vi "PythonIDE.vi"(7 "Python version":string="3.9", 9 "Processor":u16(ring) items=["SPIKE", "Pi", "Pi_ssh"], 11 "Port":string) -> ()   [LabVIEW 2020]
uses:
  <vilib>/event_ctls.llb/eventvkey.ctl
  <vilib>/Utility/miscctls.llb/LVSelectionTypeDef.ctl
  Comm_Global.vi
  <vilib>/Platform/browser.llb/Open URL in Default Browser (string).vi
panel:
  out "Text.Scroll Position":u32
  in  "Format":T1(ring)
  in  "Name":string="main.py"
  in  "Spaces":bool
  out "Shift":bool
  in  "Explorer":u16(ring) items=["Explore...", "Arm", "Backpack", "Image", "Motors", "Pinouts", "Scope", "Spatial Toolbox", "Twin"]
  in  "reconnect":bool
  out "VKey":T2
  in  "Browser":bool
  out "error IO":errorcluster
  in  "Tree":string(tree)
  in  "CtrlE":bool
  in  "Font Size":u32=12
  in  "run":bool
  in  "Save SPIKE":bool
  out "Script":string
  in  "Python Code":string
  out "Line #":string
  out "Buffer":i32(slide) scale=0.0..100000.0
  out "Graph":dbl[](graph)
  out "JPG":picture
  out "Chart":dbl[](graph)
  out "Console":string
  out "Path":path
  in  "Clear":bool
  in  "Ctrl C":bool
  in  "Save Log":bool
  in  "stop":bool
  # "PyVIEW IDE\nversion 0.1b21"
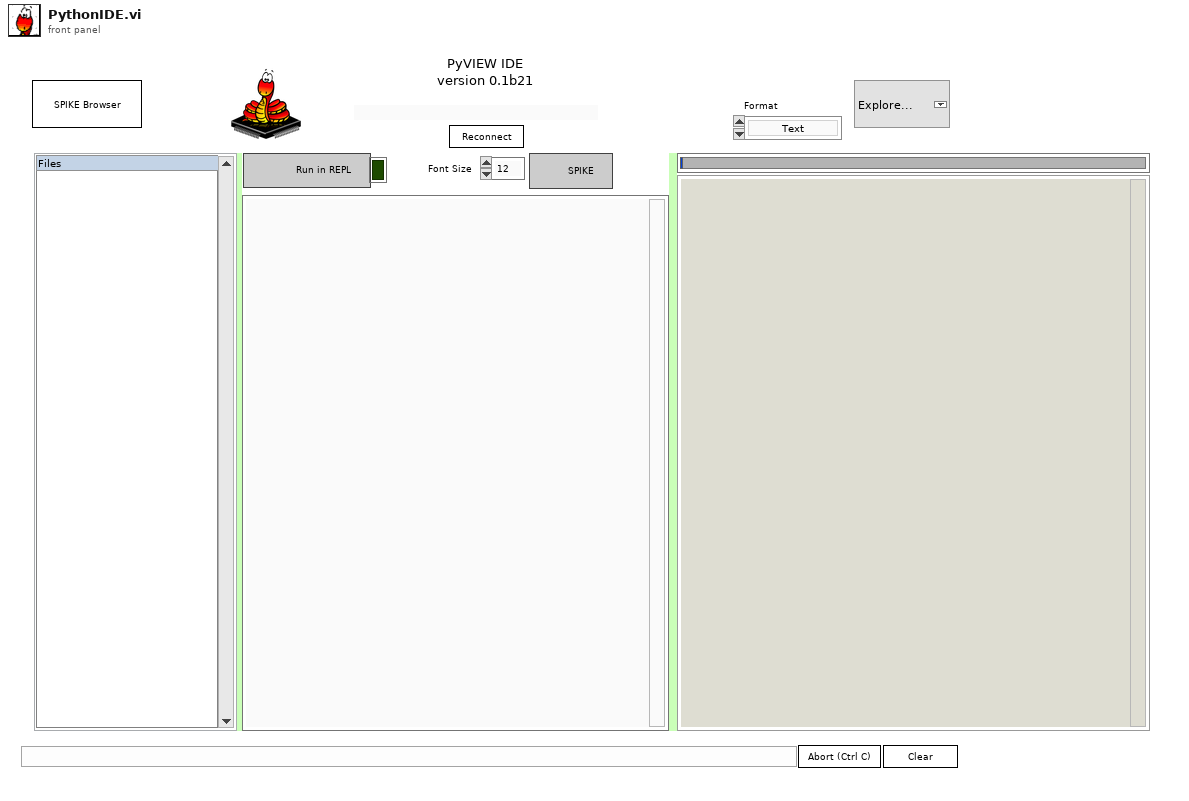
[diagram p1: front panel]
types:
  T1 = enum16{"Text", "Chart", "Waveforms", "JPEG", "Split View"}
  T2 = typedef "eventvkey.ctl" = enum16{"ASCII", "Enter", "Return", "Shift", "Ctrl", "Alt", "Cmd", "Opt", "Caps", "NumLock", "Clear", "Break", "Up", "Down", "Left", "Right", "Insert", "Delete", "Home", "End", "PageUp", "PageDown", "Escape", "Help", "Pause", "ScrollLock", "F1", "F2", "F3", "F4", "F5", "F6", "F7", "F8", "F9", "F10", "F11", "F12", "F13", "F14", "F15", "F16", "F17", "F18", "F19", "F20", "F21", "F22", "F23", "F24", "Play", "VolumeUp", "VolumeDown", "Mute", "Two Byte Char"}
  T3 = typedef "PythonCtrl.ctl" = cluster{"session":refnum<k35>, "PyPath":path, "Processor":T4}
  T4 = typedef "Processors.ctl" = enum16{"SPIKE", "Pi", "Pi_ssh", "OpenMV"}
  T5 = enum8{"Enabled", "Disabled", "Disabled and Grayed Out"}
  T6 = typedef "LVSelectionTypeDef.ctl" = cluster{"Selection Start":u32, "Selection End":u32}
  T7 = enum16{"Not data", "single values", "XY pairs", "Arrays"}
  T8 = typedef "LVPoint32TypeDef.ctl" = cluster{"Horizontal":i32, "Vertical":i32}
  T9 = typedef "Preferences.ctl" = cluster{"python":string, "arduino15":path, "arduino Lib":path, "pythonCodes":cluster{"pythonCode":path, "Color":u32}[], "FontSize":u8, "Text Colors":cluster{"Quote":u32, "function":u32, "Python":u32, "Comment":u32, "Triple Quote":u32, "Text":u32}, "Raspberry Pi":cluster{"Username":string, "password":string}}
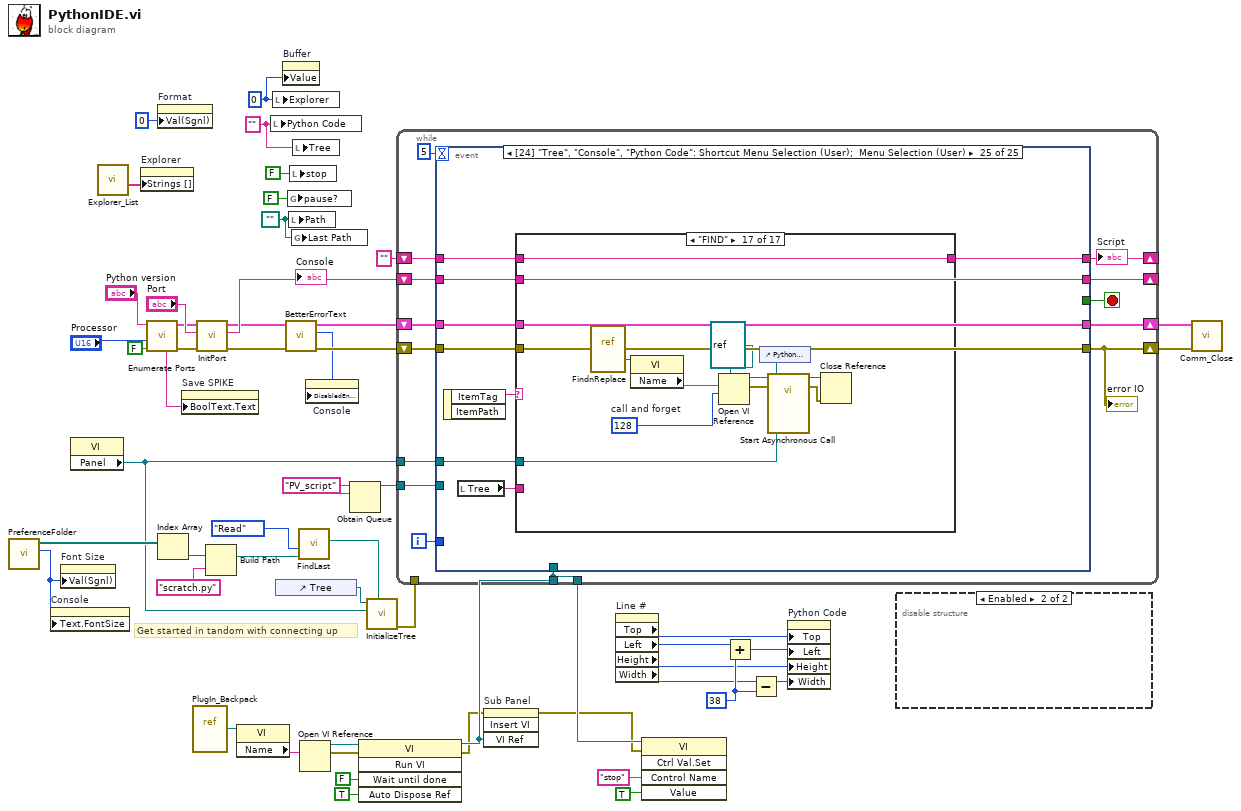
[diagram p0: block diagram]
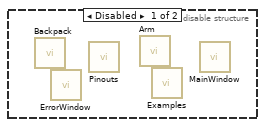
[diagram p2: hidden frame]
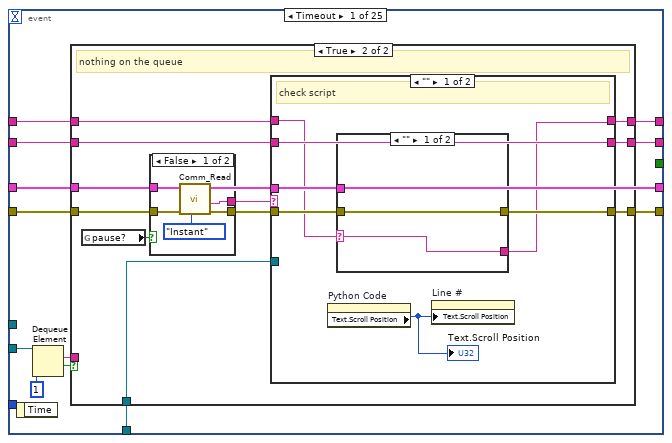
[diagram p3: hidden frame]
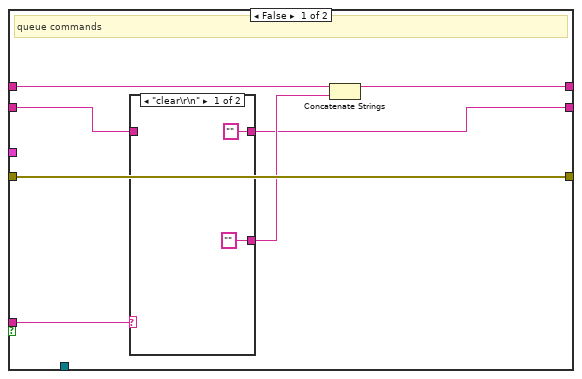
[diagram p4: hidden frame]
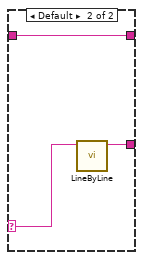
[diagram p5: hidden frame]
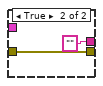
[diagram p6: hidden frame]
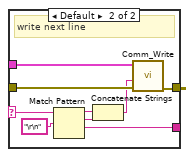
[diagram p7: hidden frame]
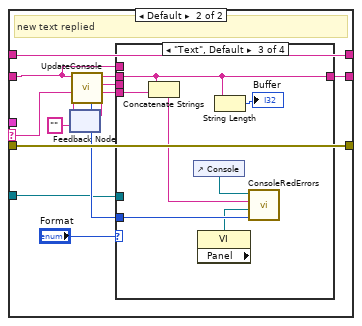
[diagram p8: hidden frame]
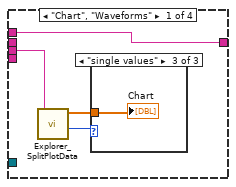
[diagram p9: hidden frame]
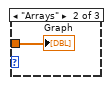
[diagram p11: hidden frame]
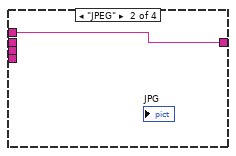
[diagram p12: hidden frame]
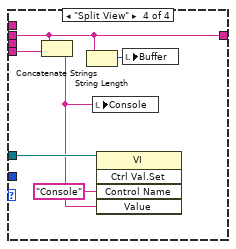
[diagram p13: hidden frame]
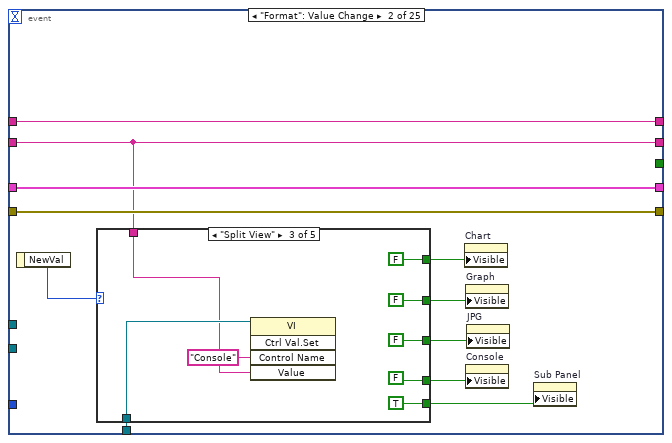
[diagram p14: hidden frame]
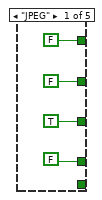
[diagram p15: hidden frame]
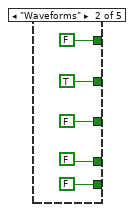
[diagram p16: hidden frame]
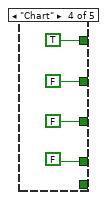
[diagram p17: hidden frame]
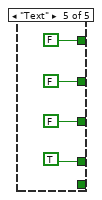
[diagram p18: hidden frame]
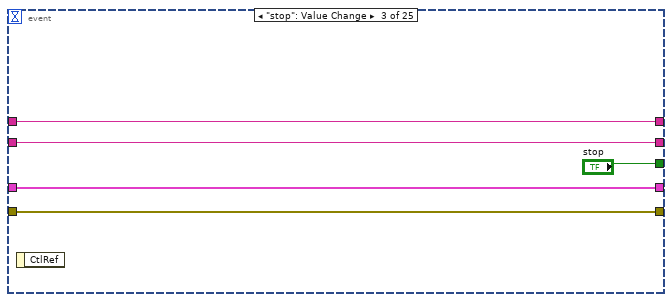
[diagram p19: hidden frame]
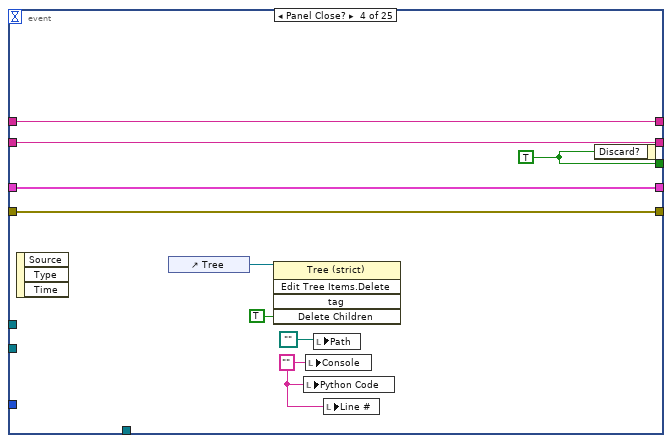
[diagram p20: hidden frame]
diagram:
  w26 = 38 ("y")
  w18 = path "" ("Path")
  w29 = 0
  w43 = "PV_script" ("name (unnamed)")
  w46 = "" ("Python Code")
  # "Get started in tandom with connecting up"
  n1 = call "PreferenceFolder.vi"() -> ("FontSize"=w16:u8, "pythonCodes"=w34:path[])  [unwired: 6 in, 4 out]
  n2 = property on="Console" class="Str"("Text.FontSize"=w16) -> ()  [unwired: 2 in, 2 out]
  n3 = property on="Font Size" class="DigNum (strict)"("Val(Sgnl)"=w16) -> ()  [unwired: 2 in, 2 out]
  n4 = property class="VI"() -> ("Panel"=w1:refnum<vi>)  [unwired: 2 in, 2 out]
  n5 = call "Explorer_List.vi"() -> ("Options"=w41:string[])  [unwired: 9 in, 2 out]
  n6 = property on="Explorer" class="Ring (strict)"("Strings []"=w41) -> ()  [unwired: 2 in, 2 out]
  n7 = call "Enumerate Ports.vi"("list?"=FALSE, "Processor"="Processor", "Python version"="Python version") -> ("error out"=w48:errorcluster, "Python"=w49:T3, "name"=w40:string)  [unwired: 4 in, 2 out]
  n8 = property on="Format" class="Enum (strict)"("Val(Sgnl)"=0) -> ()  [unwired: 2 in, 2 out]
  n9 = Index Array(array=w34) -> (element=w33:path)  [unwired: 1 in]
  n10 = property on="Save SPIKE" class="Bool"("BoolText.Text"=w40) -> ()  [unwired: 2 in, 2 out]
  n11 = vi-ref "PlugIn_Backpack.vi"() -> (w9:refnum<vi>)
  n12 = call "InitPort.vi"("error in (no error)"=w48, "Port"="Port", "Python"=w49) -> ("error out"=w15:errorcluster, "Console"=w36:string, "Python out"=w28:T3)  [unwired: 6 in]
  "Console" <- w36
  n13 = Build Path(base path=w33, name or relative path="scratch.py" ("Python Code")) -> (appended path=w32:path)
  n14 = property class="VI"(reference=w9) -> ("Name"=w7:string)  [unwired: 1 in, 2 out]
  n15 = local write "Python Code"(w46) -> ()
  n16 = local write "Explorer"(w29) -> ()
  n17 = control-ref of="Tree"() -> (w38:refnum<vi>)
  n18 = property on="Buffer" class="Slide (strict)"("Value"=w29) -> ()  [unwired: 2 in, 2 out]
  n19 = call "BetterErrorText.vi"("error in (no error)"=w15, "Python"=w28) -> ("Disabled"=w14:T5, "Python out"=w19:T3)  [unwired: 8 in]
  n20 = global write "Comm_Global.vi" "pause?"(FALSE ("pause?")) -> ()
  n21 = local write "Path"(w18) -> ()
  n22 = local write "stop"(FALSE ("stop")) -> ()
  n23 = global write "Comm_Global.vi" "Last Path"(w18) -> ()
  n24 = local write "Tree"(w46) -> ()
  n25 = call "FindLast.vi"("default"=w32, "Task"=enum16{"Save", "Read"}."Read") -> ("path"=w31:path)  [unwired: 9 in]
  n26 = Open VI Reference(vi path=w7) -> (vi reference=w11:refnum<vi>, error out=w10:errorcluster)  [unwired: 5 in]
  n27 = property on="Console" class="Str"("DisabledEnum"=w14) -> ()  [unwired: 2 in, 2 out]
  n28 = Obtain Queue(name (unnamed)=w43, element data type=w43) -> (queue out=w42:refnum<queue>)  [unwired: 3 in, 2 out]
  n29 = invoke class="VI" method="Run VI"(reference=w11, error in=w10, "Wait until done"=FALSE ("Wait Until Done"), "Auto Dispose Ref"=TRUE ("Auto Dispose Reference")) -> (reference out=w8:refnum<vi>, error out=w3:errorcluster)  [unwired: 1 in, 3 out]
  n30 = call "InitializeTree.vi"("Selected File"=w31, "Panel"=w1, "TreeControl in"=w38) -> ("error out"=w20:errorcluster)  [unwired: 8 in]
  n31 = while {
    shift-right: [w65] -> _
    shift-left: w36 -> [w66]
    shift-right: [w54] -> w44
    shift-left: w15 -> [w62]
    tunnel: w1 -> [w61]
    shift-right: [w59] -> _
    shift-left: "" -> [w60]
    tunnel: w42 -> [w57]
    shift-right: [w56] -> _
    shift-left: w19 -> [w58]
    tunnel: w20 -> [_]
    tunnel: w8 -> [w53]
    tunnel: [w53] -> w5
    i -> [w55]
    stop <- w64 stop-if-true
    n32 = event shown="[24] \"Tree\", \"Console\", \"Python Code\": Shortcut Menu Selection (User);  Menu Selection (User)" {
      selector: _ -> [_ _ _ _ _ _ _ _ _ _ _ _ _ _ _ _ _ _ _ _ _ _ _ _ _]
      dyn-events: _ -> [_ _ _ _ _ _ _ _ _ _ _ _ _ _ _ _ _ _ _ _ _ _ _ _ _]
      timeout: 5 -> [_ _ _ _ _ _ _ _ _ _ _ _ _ _ _ _ _ _ _ _ _ _ _ _ _]
      tunnel: w58 -> [w68 w171 w197 w203 w219 w224 w240 w324 w329 w338 w359 w379 w394 w407 w419 w437 w461 w472 w480 w487 w497 w503 w517 w526 w537]
      tunnel: w66 -> [w78 w161 w200 w210 w222 w231 w255 w327 w334 w347 w360 w385 w405 w411 w420 w442 w464 w475 _ w489 w500 w512 w523 w532 w536]
      tunnel: [w77 w161 w200 w210 w222 w231 w255 w327 w334 w347 w360 w385 w405 w411 w420 w442 w464 w475 w485 w489 w500 w512 w523 w532 w536] -> w65
      tunnel: [_ _ "stop" w207 _ _ _ _ _ _ _ _ _ _ _ _ _ _ _ _ _ _ _ _ _] -> w64
      tunnel: w62 -> [w73 w170 w199 w209 w221 w230 w249 w326 w333 w346 w355 w384 w406 w412 w418 w440 w462 w473 w486 w493 w502 w514 w525 w534 w539]
      tunnel: [w76 w170 w199 w209 w221 w230 w250 w326 w331 w346 w361 w384 w406 w412 w417 w440 w462 w473 w486 w493 w502 w514 w525 w534 w539] -> w54
      tunnel: w61 -> [_ _ _ _ _ _ _ _ _ w345 _ _ _ _ _ _ w460 _ _ _ _ _ _ _ w542]
      tunnel: [w75 w169 w198 w208 w220 w228 w246 w328 "" w344 w362 w386 w404 w410 w413 w441 w463 w474 w482 w492 w501 w513 w524 w533 w535] -> w59
      tunnel: w60 -> [w74 w169 w198 w208 w220 w229 w247 w328 _ w344 w362 w386 w404 w410 w414 w441 w463 w474 w484 w492 w501 w513 w524 w533 w538]
      tunnel: w57 -> [w72 _ _ _ _ _ _ _ _ _ _ _ _ _ _ _ _ _ _ _ _ _ _ _ _]
      tunnel: [w68 w171 w197 w203 w219 w224 w240 w324 w329 w338 w359 w379 w394 w407 w416 w437 w461 w472 w480 w487 w497 w503 w517 w526 w537] -> w56
      tunnel: w55 -> [_ _ _ _ _ _ _ _ _ w335 _ _ _ _ _ _ _ _ _ _ _ _ _ _ _]
      tunnel: w53 -> [w67 w162 _ _ _ _ _ _ _ _ _ _ _ _ _ _ _ _ _ _ _ _ _ _ _]
      event Timeout {
        n33 = event-data() -> ()  [unwired: 1 in, 1 out]
        n34 = Dequeue Element(queue=w72, timeout in ms (-1)=1) -> (element=w69:string, timed out?=w70:bool)  [unwired: 1 in, 2 out]
        n35 = case shown="True" w70 {
          tunnel: w78 -> [w79 w92]
          tunnel: [w80 w94] -> w77
          tunnel: [w85 w101] -> w76
          tunnel: [w83 w100] -> w75
          tunnel: w74 -> [w84 w99]
          tunnel: w73 -> [w85 w98]
          tunnel: w68 -> [_ w96]
          tunnel: w69 -> [w81 _]
          tunnel: w67 -> [_ w91]
          frame False {
            # "queue commands"
            n36 = case shown="\"clear\\r\\n\"" w81 {
              selector: w81 -> [_ w88]
              tunnel: ["" ("result string") w90] -> w82
              tunnel: ["" ("Console") w89] -> w80
              tunnel: w79 -> [_ w89]
              frame "clear\r\n" {
              }
              frame Default {
                n37 = call "LineByLine.vi"("Python Code"=w88) -> ("result string"=w90:string)  [unwired: 10 in]
              }
            }
            n38 = Concatenate Strings(w84, w82) -> (w83:string)
          }
          frame True {
            # "nothing on the queue"
            n39 = global read "Comm_Global.vi" "pause?"() -> (w95:bool)
            n40 = case shown="False" w95 {
              tunnel: w98 -> [w106 w108]
              tunnel: [w105 "" ("Text read")] -> w93
              tunnel: [w104 w108] -> w97
              tunnel: w96 -> [w103 _]
              frame False {
                n41 = call "Comm_Read.vi"("Task"=enum16{"Instant", "All"}."Instant", "error in (no error)"=w106, "Python"=w103) -> ("error out"=w104:errorcluster, "Text read"=w105:string)  [unwired: 7 in]
              }
              frame True {
              }
            }
            n42 = case shown="\"\"" w93 {
              selector: w93 -> [_ w133]
              tunnel: w92 -> [w112 w128]
              tunnel: w97 -> [w115 w140]
              tunnel: [w114 w140] -> w101
              tunnel: w99 -> [w111 w139]
              tunnel: [w110 w139] -> w100
              tunnel: w96 -> [w113 _]
              tunnel: [w112 w129] -> w94
              tunnel: w91 -> [_ w127]
              frame "" {
                # "check script"
                n43 = property on="Python Code" class="Str"() -> ("Text.Scroll Position"=w109:u32)  [unwired: 2 in, 2 out]
                "Text.Scroll Position" <- w109
                n44 = case shown="\"\"" w111 {
                  selector: w111 -> [w116 w118]
                  tunnel: [w116 w126] -> w110
                  tunnel: w115 -> [w117 w122]
                  tunnel: [w117 w121] -> w114
                  tunnel: w113 -> [_ w119]
                  frame "" {
                  }
                  frame Default {
                    # "write next line"
                    n45 = Match Pattern(string=w118, regular expression="\r\n") -> (before substring=w124:string, match substring=w123:string, after substring=w126:string)  [unwired: 1 in, 1 out]
                    n46 = Concatenate Strings(w124, w123) -> (w120:string)
                    n47 = call "Comm_Write.vi"("error in (no error)"=w122, "Text to write"=w120, "Python"=w119) -> ("error out"=w121:errorcluster)  [unwired: 8 in]
                  }
                }
                n48 = property on="Line #" class="Str"("Text.Scroll Position"=w109) -> ()  [unwired: 2 in, 2 out]
              }
              frame Default {
                # "new text replied"
                n49 = feedback #1("" ("Left over raw")) -> (w137:string)
                n50 = call "UpdateConsole.vi"("from last time raw"=w137, "New Text"=w133, "Console"=w128) -> ("Left over raw"=w138:string, "left over fixed"=w131:string, "LastFullLine"=w132:string, "Console Out"=w130:string, "cursor out"=w135:i32)  [unwired: 4 in]
                n51 = feedback-in #1(w138) -> ()
                n52 = case shown="\"Text\", Default" "Format" {
                  tunnel: w135 -> [_ _ w154 _]
                  tunnel: w132 -> [w144 _ _ _]
                  tunnel: w130 -> [_ _ w150 w159]
                  tunnel: w131 -> [_ _ w152 w160]
                  tunnel: [w141 w147 w150 w159] -> w129
                  tunnel: w128 -> [w141 w147 _ _]
                  tunnel: w127 -> [_ _ _ w156]
                  frame "Chart", "Waveforms" {
                    n53 = call "Explorer_SplitPlotData.vi"("Value"=w144) -> ("Data type"=w142:T7, "Array"=w143:dbl[])  [unwired: 9 in]
                    n54 = case shown="\"single values\"" w142 {
                      tunnel: w143 -> [_ w145 w146]
                      frame Default {
                      }
                      frame "Arrays" {
                        "Graph" <- w145
                      }
                      frame "single values" {
                        "Chart" <- w146
                      }
                    }
                  }
                  frame "JPEG" {
                  }
                  frame "Text", Default {
                    n55 = Concatenate Strings(w150, w152) -> (w151:string)
                    n56 = control-ref of="Console"() -> (w149:refnum<vi>)
                    n57 = property class="VI"() -> ("Panel"=w148:refnum<vi>)  [unwired: 2 in, 2 out]
                    n58 = String Length(string=w150) -> (length=→"Buffer":i32)
                    n59 = call "ConsoleRedErrors.vi"("Text.Selection:End"=w154, "Front Panel"=w148, "Console in"=w151, "String in"=w149) -> ()  [unwired: 6 in, 2 out]
                  }
                  frame "Split View" {
                    n60 = Concatenate Strings(w159, w160) -> (w155:string)
                    n61 = String Length(string=w159) -> (length=w158:i32)
                    n62 = local write "Console"(w155) -> ()
                    n63 = invoke class="VI" method="Ctrl Val.Set"(reference=w156, "Control Name"="Console", "Value"=w155) -> ()  [unwired: 2 in, 5 out]
                    n64 = local write "Buffer"(w158) -> ()
                  }
                }
              }
            }
          }
        }
      }
      event "Format": Value Change {
        n65 = event-data() -> ("NewVal"=w168:T1)  [unwired: 1 in]
        n66 = case shown="\"Split View\"" w168 {
          tunnel: [TRUE ("Visible") FALSE ("Visible") FALSE ("Visible") FALSE ("Visible") FALSE ("Visible")] -> w167
          tunnel: [FALSE ("Visible") TRUE ("Visible") FALSE ("Visible") FALSE ("Visible") FALSE ("Visible")] -> w166
          tunnel: [FALSE ("Visible") FALSE ("Visible") FALSE ("Visible") TRUE ("Visible") FALSE ("Visible")] -> w165
          tunnel: [FALSE ("Visible") FALSE ("Visible") FALSE ("Visible") FALSE ("Visible") TRUE ("Visible")] -> w164
          tunnel: [_ FALSE ("Visible") TRUE ("Visible") _ _] -> w163
          tunnel: w162 -> [_ _ w182 _ _]
          tunnel: w161 -> [_ _ w181 _ _]
          frame "JPEG" {
          }
          frame "Waveforms" {
          }
          frame "Split View" {
            n67 = invoke class="VI" method="Ctrl Val.Set"(reference=w182, "Control Name"="Console", "Value"=w181) -> ()  [unwired: 2 in, 5 out]
          }
          frame "Chart" {
          }
          frame "Text" {
          }
        }
        n68 = property on="Chart" class="WFChart (strict)"("Visible"=w165) -> ()  [unwired: 2 in, 2 out]
        n69 = property on="Graph" class="WFGraph (strict)"("Visible"=w166) -> ()  [unwired: 2 in, 2 out]
        n70 = property on="Console" class="Str"("Visible"=w164) -> ()  [unwired: 2 in, 2 out]
        n71 = property on="JPG" class="Pict"("Visible"=w167) -> ()  [unwired: 2 in, 2 out]
        n72 = property on="Sub Panel" class="SubPnl"("Visible"=w163) -> ()  [unwired: 2 in, 2 out]
      }
      event "stop": Value Change {
        n73 = event-data() -> ()  [unwired: 1 in, 1 out]
      }
      event Panel Close? {
        w202 = "" ("source")
        w207 = TRUE ("stop")
        n74 = event-data() -> ()  [unwired: 1 in, 3 out]
        n75 = control-ref of="Tree"() -> (w206:refnum<vi>)
        n76 = invoke on="Invoke Node" class="Tree (strict)" method="Edit Tree Items.Delete"(reference=w206, "Delete Children"=TRUE ("Delete Children?")) -> ()  [unwired: 3 in, 5 out]
        n77 = local write "Python Code"(w202) -> ()
        n78 = local write "Console"(w202) -> ()
        n79 = local write "Path"(path "") -> ()
        n80 = local write "Line #"(w202) -> ()
        n81 = event-data("Discard?"=w207) -> ()  [unwired: 1 in, 1 out]
      }
      event Pane Size; Panel Resize {
        w213 = 38 ("y")
        n82 = event-data() -> ()  [unwired: 1 in, 5 out]
        n83 = property on="Line #" class="Str"() -> ("Top"=w216:i32, "Left"=w218:i32, "Height"=w215:u32, "Width"=w214:u32)  [unwired: 2 in, 2 out]
        n84 = local read "Text.Scroll Position"() -> (w211:u32)
        n85 = Add(x=w218, y=w213) -> (x+y=w217:i32)
        n86 = Subtract(x=w214, y=w213) -> (x-y=w212:u32)
        n87 = property on="Python Code" class="Str"("Text.Scroll Position"=w211, "Top"=w216, "Left"=w217, "Height"=w215, "Width"=w212) -> ()  [unwired: 2 in, 2 out]
      }
      event "run": Value Change {
        n88 = event-data() -> ()  [unwired: 1 in, 1 out]
        n89 = local read "Processor"() -> (w225:u16)
        n90 = case shown="False" "CtrlE" {
          tunnel: [w234 w237] -> w227
          tunnel: "Python Code" -> [w233 w238]
          tunnel: w225 -> [w232 _]
          frame False {
            n91 = call "LineByLine.vi"("Processor"=w232, "Python Code"=w233) -> ("result string"=w234:string)  [unwired: 9 in]
          }
          frame True {
            n92 = Concatenate Strings("\u0005" ("string"), w238, "\u0004" ("string")) -> (w237:string)
          }
        }
        n93 = Concatenate Strings(w229, w227) -> (w228:string)
      }
      event Key Down? {
        n94 = event-data() -> ("PlatMods.Shift"=w241:bool, "PlatMods.Cmd"=w251:bool, "PlatMods.Ctrl"=w252:bool, "Char"=w253:i16, "VKey"=w254:T2)  [unwired: 1 in]
        "VKey" <- w254
        "Shift" <- w241
        n95 = property on="Python Code" class="Str"() -> ("Key Focus"=w243:bool)  [unwired: 2 in, 2 out]
        n96 = property on="Sub Panel" class="SubPnl"() -> ("Key Focus"=w239:bool)  [unwired: 2 in, 2 out]
        n97 = property on="Name" class="Str"() -> ("Key Focus"=w244:bool)  [unwired: 2 in, 2 out]
        n98 = Compound Arithmetic op=OR(w239, w243, w244) -> (w242:bool)
        n99 = case shown="False" w242 {
          tunnel: w240 -> [w264 _]
          tunnel: w254 -> [w266 _]
          tunnel: w253 -> [w265 w317]
          tunnel: w252 -> [w257 _]
          tunnel: w251 -> [w258 _]
          tunnel: [w262 w319] -> w250
          tunnel: w249 -> [w263 w319]
          tunnel: [w259 w316] -> w248
          tunnel: w247 -> [w261 w318]
          tunnel: [w260 w318] -> w246
          tunnel: w241 -> [_ w315]
          frame False {
            n100 = Or(x=w258, y=w257) -> (x .or. y?=w256:bool)
            n101 = case shown="True" w256 {
              tunnel: w266 -> [w273 _]
              tunnel: w265 -> [w272 w289]
              tunnel: w264 -> [w271 w288]
              tunnel: w263 -> [w270 w287]
              tunnel: [w268 w286] -> w262
              tunnel: w261 -> [w267 w285]
              tunnel: [w267 w284] -> w260
              tunnel: w258 -> [_ w283]
              tunnel: [_ w282] -> w259
              frame False {
                n102 = case shown="\"Right\"" w273 {
                  tunnel: w272 -> [_ _ _ _ _ w281]
                  tunnel: ["\r\n" ("replace string (\"\")") "\u001b[A" ("replace string (\"\")") "\u001b[B" ("replace string (\"\")") "\u001b[D" ("replace string (\"\")") "\u001b[C" ("replace string (\"\")") w279] -> w269
                  frame "Enter", "Return" {
                  }
                  frame "Up" {
                  }
                  frame "Down" {
                  }
                  frame "Left" {
                  }
                  frame "Right" {
                  }
                  frame Default {
                    n103 = Build Array(w281) -> (w280:i16[])
                    n104 = Byte Array To String(unsigned byte array=w280) -> (string=w279:string)
                  }
                }
                n105 = call "Comm_Write.vi"("error in (no error)"=w270, "Text to write"=w269, "Python"=w271) -> ("error out"=w268:errorcluster)  [unwired: 8 in]
              }
              frame True {
                n106 = case shown="Default" w289 {
                  selector: w289 -> [w292 _]
                  tunnel: w288 -> [w297 _]
                  tunnel: w287 -> [w296 w314]
                  tunnel: [w295 w314] -> w286
                  tunnel: w285 -> [w293 w313]
                  tunnel: [w293 w312] -> w284
                  tunnel: w283 -> [w291 _]
                  tunnel: [w290 _] -> w282
                  frame Default {
                    n107 = case shown="False" w291 {
                      tunnel: [w299 "" ("string")] -> w294
                      tunnel: w292 -> [w298 _]
                      tunnel: [_ TRUE ("Discard?")] -> w290
                      frame False {
                        # "Ctrl - clean up"
                        n108 = case shown="98" w298 {
                          tunnel: w298 -> [_ _ _ _ w305]
                          tunnel: ["\u0003" ("string") "\u0002" ("string") "\u0004" ("string") "\u0005" ("string") w304] -> w299
                          frame 67, 99 {
                          }
                          frame 98 {
                            # "Ctrl B PC"
                          }
                          frame 68, 100 {
                          }
                          frame 101 {
                            # "Ctrl E PC"
                          }
                          frame Default {
                            # "Ctrl C PC"
                            n109 = Build Array(w305) -> (w306:i16[])
                            n110 = Byte Array To String(unsigned byte array=w306) -> (string=w304:string)
                          }
                        }
                      }
                      frame True {
                        # "Cmd C/V use OS"
                      }
                    }
                    n111 = call "Comm_Write.vi"("error in (no error)"=w296, "Text to write"=w294, "Python"=w297) -> ("error out"=w295:errorcluster)  [unwired: 8 in]
                  }
                  frame 22, 118 {
                    # "paste"
                    n112 = invoke class="App" method="Clipboard.Read"() -> ("Read Clipbrd"=w311:string)  [unwired: 3 in, 2 out]
                    n113 = local read "Processor"() -> (w309:u16)
                    n114 = call "LineByLine.vi"("Processor"=w309, "Python Code"=w311) -> ("result string"=w310:string)  [unwired: 9 in]
                    n115 = Concatenate Strings(w313, w310) -> (w312:string)
                  }
                }
              }
            }
          }
          frame True {
            n116 = case shown="9" w317 {
              tunnel: [TRUE ("Discard?") _] -> w316
              tunnel: w315 -> [_ w322]
              frame 0, Default {
              }
              frame 9 {
                # "Tab key"
                n117 = control-ref of="Python Code"() -> (w323:refnum<vi>)
                n118 = call "Tab_In_Out.vi"("Shift?"=w322, "String in"=w323) -> ("result string"=w321:string)  [unwired: 9 in]
                n119 = property on="Python Code" class="Str"("Val(Sgnl)"=w321) -> ()  [unwired: 2 in, 2 out]
              }
            }
          }
        }
        n120 = Not(x=w248) -> (.not. x?=w245:bool)
        n121 = event-data("Discard?"=w245) -> ()  [unwired: 1 in, 1 out]
      }
      event Key Up {
        n122 = event-data() -> ()  [unwired: 1 in, 8 out]
        n123 = local write "Shift"(FALSE ("Shift")) -> ()
      }
      event "Ctrl C": Value Change {
        n124 = event-data() -> ()  [unwired: 1 in, 1 out]
        n125 = call "Comm_Write.vi"("error in (no error)"=w333, "Text to write"="\u0003\r\n\r\n" ("function name"), "Python"=w329) -> ("error out"=w331:errorcluster)  [unwired: 8 in]
      }
      event "Python Code": Value Change {
        n126 = event-data() -> ()  [unwired: 1 in, 1 out]
        n127 = local read "VKey"() -> (w342:T2)
        n128 = case shown="Default" w342 {
          tunnel: [FALSE TRUE] -> w341
          frame Default {
          }
          frame "Enter", "Return" {
          }
        }
        n129 = control-ref of="Python Code"() -> (w343:refnum<vi>)
        n130 = call "Color_Assign.vi"("Add Spaces?"=w341, "Front Panel"=w345, "Code"=w343) -> ("Value"=w337:string)  [unwired: 8 in]
        n131 = call "BuildLineNumbers.vi"("Python Code"=w337) -> ("String"=→"Line #":string)  [unwired: 10 in]
        n132 = property on="Python Code" class="Str"() -> ("DisabledEnum"=w339:T5)  [unwired: 2 in, 2 out]
        n133 = local read "Tree"() -> (w340:string)
        n134 = case shown="\"Enabled\"" w339 {
          tunnel: w337 -> [_ w351]
          tunnel: w340 -> [_ w350]
          tunnel: w335 -> [_ w348]
          frame Default {
          }
          frame "Enabled" {
            n135 = case shown="0..5" w348 {
              frame Default {
              }
              frame 0..5 {
                n136 = property on="Ctrl C" class="Bool"("Key Focus"=TRUE) -> ()  [unwired: 2 in, 2 out]
              }
            }
            n137 = String To Path(string=w350) -> (path=w349:path)
            n138 = Write to Text File(file (use dialog)=w349, text=w351) -> ()  [unwired: 2 in, 3 out]
          }
        }
      }
      event "Save SPIKE": Value Change {
        n139 = event-data() -> ()  [unwired: 1 in, 3 out]
        n140 = local read "Tree"() -> (w358:string)
        n141 = String To Path(string=w358) -> (path=w357:path)
        n142 = Strip Path(path=w357) -> (name=w356:string)  [unwired: 1 out]
        n143 = case shown="No Error" w355 {
          selector: w355 -> [w363 w378]
          tunnel: [w370 w378] -> w361
          tunnel: w360 -> [w369 _]
          tunnel: w359 -> [w365 _]
          tunnel: w356 -> [w364 _]
          frame No Error {
            n144 = call "AskRename.vi"("Prompt"="Name on Spike?", "name"=w364) -> ("OK?"=w367:bool, "name 2"=w368:string)  [unwired: 8 in]
            n145 = case shown="True" w367 {
              tunnel: w365 -> [_ w377]
              tunnel: w363 -> [w371 w376]
              tunnel: [w371 w375] -> w370
              tunnel: w369 -> [_ w373]
              tunnel: w368 -> [_ w372]
              frame False {
              }
              frame True {
                n146 = local read "Python Code"() -> (w374:string)
                n147 = call "ReadFileDialog.vi"("File Text"=w374, "error in (no error)"=w376, "File name"=w372, "Console in"=w373, "Python in"=w377) -> ("error out"=w375:errorcluster)  [unwired: 5 in, 1 out]
              }
            }
          }
          frame Error {
          }
        }
      }
      event "Explorer": Value Change {
        n148 = event-data() -> ("NewVal"=w381:u16)  [unwired: 1 in, 1 out]
        n149 = property on="Explorer" class="Ring (strict)"() -> ("Strings []"=w382:string[])  [unwired: 2 in, 2 out]
        n150 = Index Array(array=w382, index=w381) -> (element=w380:string)
        n151 = case shown="Default" w381 {
          tunnel: w380 -> [_ w391]
          frame 0 {
          }
          frame Default {
            n152 = local read "Shift"() -> (w390:bool)
            n153 = Select(t=enum16{"run", "open"}."open" ("Task"), s=w390, f=enum16{"run", "open"}."run" ("Task")) -> (s? t:f=w387:enum16{"run", "open"})
            n154 = control-ref of="Console"() -> (w392:refnum<vi>)
            n155 = call "Explore_Open.vi"("Task"=w387, "Name"=w391, "String in"=w392) -> ()  [unwired: 9 in]
          }
        }
        n156 = local write "Explorer"(0) -> ()
      }
      event "Browser": Value Change {
        w402 = 128  # call and forget
        n157 = event-data() -> ()  [unwired: 1 in, 3 out]
        n158 = vi-ref "Examples.vi"() -> (w399:refnum<vi>)
        n159 = property class="VI"(reference=w399) -> ("Name"=w400:string)  [unwired: 1 in, 2 out]
        n160 = local read "Python version"() -> (w393:string)
        n161 = local read "Port"() -> (w398:string)
        n162 = Open VI Reference(type specifier VI Refnum (for type only)=refnum<vi> refnum, vi path=w400, options=w402) -> (vi reference=w403:refnum<vi>, error out=w395:errorcluster)  [unwired: 3 in]
        n163 = call-by-ref "Start Asynchronous Call"(reference=w403, error in=w395, "Python version"=w393, "Python"=w394, "Port"=w398) -> (reference out=w396:refnum<vi>, error out=w397:errorcluster)  [unwired: 9 in]
        n164 = Close Reference(reference=w396, error in (no error)=w397) -> ()  [unwired: 1 out]
      }
      event "Spaces": Value Change {
        n165 = event-data() -> ()  [unwired: 1 in, 3 out]
        n166 = property on="Python Code" class="Str"() -> ("Value"=w408:string)  [unwired: 2 in, 2 out]
        n167 = call "CleanUp.vi"("Python Code"=w408) -> ("spreadsheet string"=w409:string)  [unwired: 10 in]
        n168 = property on="Python Code" class="Str"("Val(Sgnl)"=w409) -> ()  [unwired: 2 in, 2 out]
      }
      event "reconnect": Value Change {
        n169 = event-data() -> ()  [unwired: 1 in, 3 out]
        n170 = flat-sequence {
          tunnel: w419 -> [w421]
          tunnel: w418 -> [w422]
          tunnel: [w426] -> w417
          tunnel: [w425] -> w416
          frame #0 {
            n171 = call "Comm_Close.vi"("error in (no error)"=w422, "Python in"=w421) -> ()  [unwired: 9 in, 1 out]
          }
          frame #1 {
            n172 = Wait (ms)(milliseconds to wait=u32 10) -> ()  [unwired: 1 out]
          }
          frame #2 {
            n173 = local read "Python version"() -> (w429:string)
            n174 = local read "Processor"() -> (w428:u16)
            n175 = call "Enumerate Ports.vi"("Processor"=w428, "Python version"=w429) -> ("Python"=w430:T3)  [unwired: 5 in, 4 out]
            n176 = local read "Port"() -> (w431:string)
            n177 = call "InitPort.vi"("Port"=w431, "Python"=w430) -> ("error out"=w426:errorcluster, "Python out"=w427:T3)  [unwired: 7 in, 1 out]
            n178 = call "BetterErrorText.vi"("error in (no error)"=w426, "Python"=w427) -> ("Disabled"=w424:T5, "Python out"=w425:T3)  [unwired: 8 in]
            n179 = property on="Console" class="Str"("DisabledEnum"=w424) -> ()  [unwired: 2 in, 2 out]
          }
        }
        n180 = Concatenate Strings(w414, "\r\n" ("string")) -> (w413:string)
      }
      event "Tree": Value Change {
        # "need this to keep\nfrom adding spaces"
        # "rebuild tree and load new file"
        n181 = event-data() -> ()  [unwired: 1 in, 3 out]
        n182 = String To Path(string="Tree") -> (path=w434:path)
        "Path" <- w434
        n183 = global write "Comm_Global.vi" "Last Path"(w434) -> ()
        n184 = local write "VKey"(eventvkey."ASCII" ("VKey")) -> ()
        n185 = Read from Text File(file (use dialog)=w434) -> (text=w439:string, error out=w438:errorcluster)  [unwired: 3 in, 2 out]
        n186 = case shown="No Error" w438 {
          tunnel: w439 -> [w453 _]
          tunnel: "Tree" -> [w451 _]
          tunnel: [TRUE ("enabled") FALSE ("enabled")] -> w433
          frame No Error {
            n187 = call "FindLast.vi"("Task"=enum16{"Save", "Read"}."Save", "Tree"=w451) -> ()  [unwired: 9 in, 1 out]
            n188 = property on="Python Code" class="Str"("Val(Sgnl)"=w453, "DisabledEnum"=T5."Enabled" ("Disabled"), "Text.Selection"=T6 {"Selection Start"=0, "Selection End"=0}, "Text.Scroll Position"=u32 0, "Key Focus"=FALSE) -> ()  [unwired: 2 in, 2 out]
          }
          frame Error {
            n189 = property on="Python Code" class="Str"("Val(Sgnl)"="" ("Python Code"), "DisabledEnum"=T5."Disabled and Grayed Out" ("Disabled")) -> ()  [unwired: 2 in, 2 out]
          }
        }
        n190 = for {
          tunnel: w433 -> [w444]
          tunnel: string[] ["WINDOW", "OPEN", "RENAME", "DUPLICATE", "DELETE_TREE", "SAVEAS_TREE", "SPACES", "RUN"] -> [w443] mode=indexing
          n191 = Current VI's Menubar() -> (w445:refnum<k9>)
          n192 = Set Menu Item Info(7:w443, 9:w444, 11:w445) -> ()  [unwired: 4 in, 2 out]
        }
      }
      event "Tree": Double Click {
        # "rebuild tree and load new file"
        n193 = event-data() -> ()  [unwired: 1 in, 1 out]
        n194 = local read "Tree"() -> (w458:string)
        n195 = String To Path(string=w458) -> (path=w459:path)
        n196 = Read from Text File(file (use dialog)=w459) -> (error out=w457:errorcluster)  [unwired: 3 in, 3 out]
        n197 = case shown="No Error" w457 {
          tunnel: w460 -> [w466 _]
          tunnel: w458 -> [w465 _]
          frame No Error {
            n198 = control-ref of="Tree"() -> (w467:refnum<vi>)
            n199 = call "Tree_Rename.vi"("Tree in"=w465, "Panel"=w466, "TreeControl in"=w467) -> ()  [unwired: 9 in]
          }
          frame Error {
          }
        }
      }
      event "Tree": Drop {
        # "Dragging"
        n200 = event-data() -> ("Coords"=w470:T8)  [unwired: 1 in]
        n201 = invoke on="Tree" class="Tree (strict)" method="Point To Row Column"("Point"=w470) -> ("InBounds"=w468:bool, "Tag"=w469:string)  [unwired: 7 in, 6 out]
        n202 = case shown="True" w468 {
          tunnel: w469 -> [_ w477]
          frame False {
          }
          frame True {
            # "original path"
            # "tag where released"
            n203 = local read "Tree"() -> (w476:string)
            n204 = flat-sequence {
              tunnel: w476 -> [_]
              tunnel: w477 -> [_]
              frame #0 {
              }
            }
          }
        }
        n205 = event-data("Accepted?"=FALSE) -> ()  [unwired: 1 in, 1 out]
      }
      event "Clear": Value Change {
        w485 = ""
        n206 = event-data() -> ()  [unwired: 1 in, 3 out]
        n207 = Concatenate Strings(w484, "\r\n" ("string")) -> (w482:string)
        n208 = local write "Graph"(dbl[] [] ("Graph")) -> ()
        n209 = property on="Chart" class="WFChart (strict)"("History Data"=dbl[] []) -> ()  [unwired: 2 in, 2 out]
        n210 = local write "Console"(w485) -> ()
        n211 = local write "Buffer"(0) -> ()
      }
      event "Save Log": Value Change {
        n212 = event-data() -> ()  [unwired: 1 in, 3 out]
        n213 = call "File Dialog3"("default name"="log.txt") -> ("selected path"=w488:path, "error out"=w490:errorcluster)  [unwired: 11 in, 2 out]
        n214 = case shown="No Error" w490 {
          tunnel: w489 -> [w495 _]
          tunnel: w488 -> [w494 _]
          frame No Error {
            n215 = Write to Text File(file (use dialog)=w494, text=w495) -> ()  [unwired: 2 in, 3 out]
          }
          frame Error {
          }
        }
      }
      event "Font Size": Value Change {
        n216 = event-data() -> ()  [unwired: 1 in, 3 out]
        n217 = call "Preferences.vi"() -> ("Preferences out"=w498:T9)  [unwired: 10 in, 1 out]
        n218 = Bundle By Name(cluster=w498, "FontSize"="Font Size") -> (w499:T9)
        n219 = property on="Python Code" class="Str"("Text.FontSize"="Font Size") -> ()  [unwired: 2 in, 2 out]
        n220 = call "Preferences.vi"("Preferences in"=w499) -> ()  [unwired: 9 in, 2 out]
        n221 = property on="Console" class="Str"("Text.FontSize"="Font Size") -> ()  [unwired: 2 in, 2 out]
      }
      event "Tree": Shortcut Menu Activation? {
        n222 = event-data() -> ("MenuRef"=w508:refnum<k9>)  [unwired: 1 in]
        n223 = local read "Tree"() -> (w506:string)
        n224 = String To Path(string=w506) -> (path=w505:path)
        n225 = call <vilib>:"Get File Extension.vi"("file"=w505) -> ("lowercase file extension"=w504:string)  [unwired: 6 in, 4 out]
        n226 = case shown="\"py\"" w504 {
          tunnel: [string[] ["Open in Finder"] ("L10n_Parent Menus") string[] ["Open in Finder", "Open in new window", "Duplicate", "Rename...", "Save As...", "Delete"] ("L10n_Parent Menus")] -> w507
          frame Default {
          }
          frame "py" {
          }
        }
        n227 = Delete Menu Items(9:w508) -> (0:w511:errorcluster, 3:w510:refnum<k9>)  [unwired: 3 in]
        n228 = Insert Menu Items(6:w511, 7:string[] ["OPEN", "WINDOW", "DUPLICATE", "RENAME", "SAVEAS_TREE", "DELETE_TREE", "COPY", "MOVE"], 8:w507, 9:w510) -> ()  [unwired: 2 in, 3 out]
        n229 = event-data() -> ()  [unwired: 2 in, 1 out]
      }
      event "Console": Shortcut Menu Activation? {
        n230 = event-data() -> ("MenuRef"=w519:refnum<k9>)  [unwired: 1 in]
        n231 = Delete Menu Items(9:w519) -> (0:w522:errorcluster, 3:w521:refnum<k9>)  [unwired: 3 in]
        n232 = Insert Menu Items(6:w522, 7:string[] ["CTRLC", "CLEAR", "SAVEAS", "ERROR"], 8:string[] ["Ctrl C", "Clear", "Save As...", "Traceback Error"] ("L10n_Parent Menus"), 9:w521) -> ()  [unwired: 2 in, 3 out]
        n233 = event-data() -> ()  [unwired: 2 in, 1 out]
      }
      event "Python Code": Shortcut Menu Activation? {
        n234 = event-data() -> ("MenuRef"=w528:refnum<k9>)  [unwired: 1 in]
        n235 = Delete Menu Items(9:w528) -> (0:w531:errorcluster, 3:w530:refnum<k9>)  [unwired: 3 in]
        n236 = Insert Menu Items(6:w531, 7:string[] ["SPACES", "RUN", "SAVEAS_CODE"], 8:string[] ["Check Spaces", "Run in REPL", "Save As..."] ("L10n_Parent Menus"), 9:w530) -> ()  [unwired: 2 in, 3 out]
        n237 = event-data() -> ()  [unwired: 2 in, 1 out]
      }
      event "Tree", "Console", "Python Code": Shortcut Menu Selection (User); Menu Selection (User) {
        n238 = event-data() -> ("ItemTag"=w540:string)  [unwired: 1 in, 1 out]
        n239 = local read "Tree"() -> (w541:string)
        n240 = case shown="\"FIND\"" w540 {
          tunnel: w542 -> [_ w551 _ w574 w586 w593 w603 w615 _ _ _ _ _ _ _ _ w666]
          tunnel: w541 -> [_ w546 w560 w572 w576 w591 w595 w609 w633 _ _ _ _ _ _ _ _]
          tunnel: w539 -> [_ _ _ _ _ _ _ _ _ _ w642 _ _ _ _ _ _]
          tunnel: w538 -> [w543 w545 w559 w571 w575 w590 w594 w608 w622 w634 _ w644 w647 w649 w657 w661 w675]
          tunnel: w537 -> [_ _ _ _ _ _ _ _ _ _ w641 _ _ _ _ _ _]
          tunnel: w536 -> [_ _ _ _ _ _ _ _ _ _ _ _ w648 _ _ _ _]
          tunnel: [w543 w545 w559 w571 w575 w590 w594 w608 w622 w634 "" w644 w647 w649 w657 w660 w675] -> w535
          frame Default {
          }
          frame "NEW" {
            n241 = String To Path(string=w546) -> (path=w550:path)
            n242 = Strip Path(path=w550) -> (stripped path=w549:path)  [unwired: 1 out]
            n243 = call "File Dialog5"("start path"=w549, "default name"="untitled.py") -> ("selected path"=w547:path, "error out"=w548:errorcluster)  [unwired: 10 in, 2 out]
            n244 = case shown="No Error" w548 {
              tunnel: w550 -> [_ _]
              tunnel: w547 -> [w557 _]
              tunnel: w551 -> [w555 _]
              frame No Error {
                n245 = control-ref of="Tree"() -> (w556:refnum<vi>)
                n246 = call "CheckForExtension.vi"("selected path"=w557) -> ("dup file"=w554:path)  [unwired: 10 in]
                n247 = Write to Text File(file (use dialog)=w554, text="") -> (error out=w553:errorcluster)  [unwired: 2 in, 2 out]
                n248 = call "InitializeTree.vi"("Selected File"=w554, "error in (no error)"=w553, "Panel"=w555, "TreeControl in"=w556) -> ()  [unwired: 7 in, 1 out]
              }
              frame Error {
              }
            }
          }
          frame "OPEN" {
            n249 = String To Path(string=w560) -> (path=w562:path)
            n250 = call <vilib>:"Get File Extension.vi"("file"=w562) -> ("lowercase file extension"=w561:string)  [unwired: 6 in, 4 out]
            n251 = case shown="\"py\"" w561 {
              tunnel: [w568 w570] -> w558
              tunnel: w562 -> [w568 w569]
              frame Default {
              }
              frame "py" {
                n252 = Strip Path(path=w569) -> (stripped path=w570:path)  [unwired: 1 out]
              }
            }
            n253 = disable-structure shown="TARGET_TYPE==Windows" {
              disable-tunnel: w558 -> [w564 w565]
              frame condition #0 (active) {
                n254 = call <vilib>:"Path to URL.vi"("path"=w564) -> ("url"=w563:string)
                n255 = call-poly <vilib>:"Open URL in Default Browser.vi"("URL"=w563) -> ()  [unwired: 5 in, 2 out]
              }
              frame condition #1 {
                n256 = Format Into String(format string="cmd /c explorer.exe \"%s\"", w565) -> (resulting string=w567:string)  [unwired: 2 in, 1 out]
                n257 = call <vilib>:"System Exec.vi"("command line"=w567) -> ()  [unwired: 7 in, 4 out]
              }
            }
          }
          frame "RENAME" {
            n258 = control-ref of="Tree"() -> (w573:refnum<vi>)
            n259 = call "Tree_Rename.vi"("Tree in"=w572, "Panel"=w574, "TreeControl in"=w573) -> ()  [unwired: 9 in]
          }
          frame "DUPLICATE" {
            n260 = String To Path(string=w576) -> (path=w588:path)
            n261 = Strip Path(path=w588) -> (stripped path=w587:path, name=w582:string)
            n262 = Search/Split String(string=w582, search string/char (-)=".py") -> (substring before match=w580:string, match + rest of string=w579:string)  [unwired: 1 in, 1 out]
            n263 = Concatenate Strings(w580, "(1)" ("search string/char (-)"), w579) -> (w578:string)
            n264 = Build Path(base path=w587, name or relative path=w578) -> (appended path=w583:path)
            n265 = control-ref of="Tree"() -> (w585:refnum<vi>)
            n266 = Copy(10:w583, 11:w588) -> (0:w584:errorcluster)  [unwired: 3 in, 2 out]
            n267 = call "InitializeTree.vi"("Selected File"=w583, "error in (no error)"=w584, "Panel"=w586, "TreeControl in"=w585) -> ()  [unwired: 7 in, 1 out]
          }
          frame "RELOAD" {
            n268 = String To Path(string=w591) -> (path=w589:path)
            n269 = control-ref of="Tree"() -> (w592:refnum<vi>)
            n270 = call "InitializeTree.vi"("Selected File"=w589, "Panel"=w593, "TreeControl in"=w592) -> ()  [unwired: 8 in, 1 out]
          }
          frame "DELETE_TREE" {
            n271 = String To Path(string=w595) -> (path=w601:path)
            n272 = Strip Path(path=w601) -> (name=w600:string)  [unwired: 1 out]
            n273 = Format Into String(format string="Are you sure you want to delete the file:  %s?", w600) -> (resulting string=w599:string)  [unwired: 2 in, 1 out]
            n274 = Two Button Dialog(message=w599, 1:"Delete" ("T button name (\"OK\")"), 2:"Cancel" ("T button name (\"OK\")")) -> (T button?=w602:bool)
            n275 = case shown="False" w602 {
              tunnel: w601 -> [w607 _]
              tunnel: w603 -> [w604 _]
              frame False {
                n276 = Delete(path (use dialog)=w607) -> (error out=w605:errorcluster)  [unwired: 4 in, 2 out]
                n277 = control-ref of="Tree"() -> (w606:refnum<vi>)
                n278 = call "InitializeTree.vi"("error in (no error)"=w605, "Panel"=w604, "TreeControl in"=w606) -> ()  [unwired: 8 in, 1 out]
              }
              frame True {
              }
            }
          }
          frame "SAVEAS_TREE" {
            n279 = String To Path(string=w609) -> (path=w613:path)
            n280 = Strip Path(path=w613) -> (stripped path=w612:path, name=w614:string)
            n281 = call "File Dialog4"("start path"=w612, "default name"=w614) -> ("selected path"=w610:path, "error out"=w611:errorcluster)  [unwired: 10 in, 2 out]
            n282 = case shown="No Error" w611 {
              tunnel: w613 -> [_ _]
              tunnel: w610 -> [w621 _]
              tunnel: w615 -> [w619 _]
              frame No Error {
                n283 = control-ref of="Tree"() -> (w620:refnum<vi>)
                n284 = local read "Python Code"() -> (w618:string)
                n285 = call "CheckForExtension.vi"("selected path"=w621) -> ("dup file"=w617:path)  [unwired: 10 in]
                n286 = Write to Text File(file (use dialog)=w617, text=w618) -> (error out=w616:errorcluster)  [unwired: 2 in, 2 out]
                n287 = call "InitializeTree.vi"("Selected File"=w617, "error in (no error)"=w616, "Panel"=w619, "TreeControl in"=w620) -> ()  [unwired: 7 in, 1 out]
              }
              frame Error {
              }
            }
          }
          frame "WINDOW" {
            w625 = 128  # call and forget
            n288 = String To Path(string=w633) -> (path=w624:path)
            n289 = vi-ref "MainWindow.vi"() -> (w629:refnum<vi>)
            n290 = property class="VI"(reference=w629) -> ("Name"=w628:string)  [unwired: 1 in, 2 out]
            n291 = Open VI Reference(type specifier VI Refnum (for type only)=refnum<vi> refnum, vi path=w628, options=w625) -> (vi reference=w627:refnum<vi>, error out=w632:errorcluster)  [unwired: 3 in]
            n292 = call-by-ref "Start Asynchronous Call"(reference=w627, error in=w632, "Path"=w624) -> (reference out=w631:refnum<vi>, error out=w630:errorcluster)  [unwired: 11 in]
            n293 = property on="Tree" class="Tree (strict)"("Val(Sgnl)"="" ("Value (Signaling)")) -> ()  [unwired: 2 in, 2 out]
            n294 = Close Reference(reference=w631, error in (no error)=w630) -> ()  [unwired: 1 out]
          }
          frame "SAVEAS" {
            n295 = call "File Dialog"("default name"="log.txt") -> ("selected path"=w636:path, "error out"=w637:errorcluster)  [unwired: 11 in, 2 out]
            n296 = case shown="No Error" w637 {
              tunnel: w636 -> [w638 _]
              frame No Error {
                n297 = local read "Console"() -> (w639:string)
                n298 = Write to Text File(file (use dialog)=w638, text=w639) -> ()  [unwired: 2 in, 3 out]
              }
              frame Error {
              }
            }
          }
          frame "CTRLC" {
            n299 = call "Comm_Write.vi"("error in (no error)"=w642, "Text to write"="\u0003\r\n\r\n" ("function name"), "Python"=w641) -> ()  [unwired: 8 in, 1 out]
          }
          frame "CLEAR" {
            n300 = local write "Console"("") -> ()
            n301 = local write "Buffer"(0) -> ()
          }
          frame "ERROR" {
            n302 = call "ErrorWindow.vi"("Console in"=w648) -> ()  [unwired: 10 in]
          }
          frame "SAVEAS_CODE" {
            n303 = local read "Path"() -> (w652:path)
            n304 = Strip Path(path=w652) -> (stripped path=w651:path, name=w650:string)
            n305 = call "File Dialog2"("start path"=w651, "default name"=w650) -> ("selected path"=w653:path, "error out"=w654:errorcluster)  [unwired: 10 in, 2 out]
            n306 = case shown="No Error" w654 {
              tunnel: w653 -> [w655 _]
              frame No Error {
                n307 = local read "Python Code"() -> (w656:string)
                n308 = Write to Text File(file (use dialog)=w655, text=w656) -> ()  [unwired: 2 in, 3 out]
              }
              frame Error {
              }
            }
          }
          frame "SPACES" {
            n309 = property on="Python Code" class="Str"() -> ("Value"=w658:string)  [unwired: 2 in, 2 out]
            n310 = call "CleanUp.vi"("Python Code"=w658) -> ("spreadsheet string"=w659:string)  [unwired: 10 in]
            n311 = property on="Python Code" class="Str"("Val(Sgnl)"=w659) -> ()  [unwired: 2 in, 2 out]
          }
          frame "RUN" {
            n312 = local read "Python Code"() -> (w662:string)
            n313 = local read "Processor"() -> (w663:u16)
            n314 = call "LineByLine.vi"("Processor"=w663, "Python Code"=w662) -> ("result string"=w664:string)  [unwired: 9 in]
            n315 = Concatenate Strings(w661, w664) -> (w660:string)
          }
          frame "FIND" {
            w667 = 128  # call and forget
            n316 = vi-ref "FindnReplace.vi"() -> (w672:refnum<vi>)
            n317 = property class="VI"(reference=w672) -> ("Name"=w673:string)  [unwired: 1 in, 2 out]
            n318 = Open VI Reference(type specifier VI Refnum (for type only)=refnum<vi> refnum, vi path=w673, options=w667) -> (vi reference=w674:refnum<vi>, error out=w669:errorcluster)  [unwired: 3 in]
            n319 = control-ref of="Python Code"() -> (w665:refnum<vi>)
            n320 = call-by-ref "Start Asynchronous Call"(reference=w674, error in=w669, "Front Panel"=w666, "Python Code"=w665) -> (reference out=w670:refnum<vi>, error out=w671:errorcluster)  [unwired: 10 in]
            n321 = Close Reference(reference=w670, error in (no error)=w671) -> ()  [unwired: 1 out]
          }
        }
      }
    }
    "Script" <- w59
    "error IO" <- w54
  }
  n322 = invoke on="Sub Panel" class="SubPnl" method="Insert VI"(error in=w3, "VI Ref"=w8) -> (error out=w2:errorcluster)  [unwired: 2 in, 3 out]
  n323 = property on="Line #" class="Str"() -> ("Top"=w23:i32, "Left"=w21:i32, "Height"=w24:u32, "Width"=w25:u32)  [unwired: 2 in, 2 out]
  n324 = invoke class="VI" method="Ctrl Val.Set"(reference=w5, error in=w2, "Control Name"="stop", "Value"=TRUE ("Auto Dispose Reference")) -> ()  [unwired: 1 in, 5 out]
  n325 = Add(x=w21, y=w26) -> (x+y=w22:i32)
  n326 = Subtract(x=w25, y=w26) -> (x-y=w27:u32)
  n327 = property on="Python Code" class="Str"("Top"=w23, "Left"=w22, "Height"=w24, "Width"=w27) -> ()  [unwired: 2 in, 2 out]
  n328 = disable-structure shown="Enabled" {
    frame Disabled {
      n329 = call "Backpack.vi"() -> ()  [unwired: 12 in]
      n330 = call "ErrorWindow.vi"() -> ()  [unwired: 11 in]
      n331 = call "Pinouts.vi"() -> ()  [unwired: 12 in]
      n332 = call "Arm.vi"() -> ()  [unwired: 12 in]
      n333 = call "Examples.vi"() -> ()  [unwired: 12 in]
      n334 = call "MainWindow.vi"() -> ()  [unwired: 12 in]
    }
    frame Enabled {
    }
  }
  n335 = call "Comm_Close.vi"("error in (no error)"=w44, "Python in"=w19) -> ()  [unwired: 9 in, 1 out]
